vi "Has Trailing Slash.vi"(11 "Path In":string) -> (3 "Path":string, 5 "Trailing Slash?":bool)   [LabVIEW 2020, in "Stream.lvlib"]
uses:
  Stream.lvlib
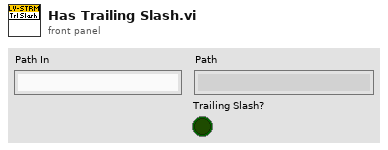
[diagram p1: front panel]
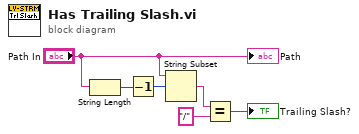
[diagram p0: block diagram]
diagram:
  n1 = String Length(string="Path In") -> (length=w6:i32)
  n2 = Decrement(x=w6) -> (x-1=w5:i32)
  n3 = String Subset(string="Path In", offset (0)=w5) -> (substring=w4:string)  [unwired: 1 in]
  n4 = Equal?(x=w4, y="/") -> (x = y?=→"Trailing Slash?":bool)
  "Path" <- "Path In"
